vi "SetOutputVoltage.vi"(8 "error in (no error)":errorcluster, 10 "Voltage":dbl, 11 "RMXPowerSupply in":refnum<class "RMXPowerSupply.lvclass">) -> (0 "error out":errorcluster, 3 "RMXPowerSupply out":refnum<class "RMXPowerSupply.lvclass">)   [LabVIEW 2023, in "RMXPowerSupply.lvclass"]
uses:
  RMXPowerSupply.lvclass
  RMXPowerSupply.lvclass/RMXPowerSupply.ctl
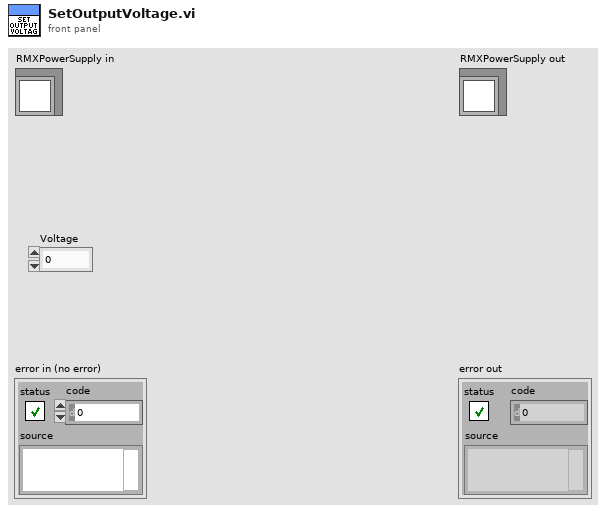
[diagram p1: front panel]
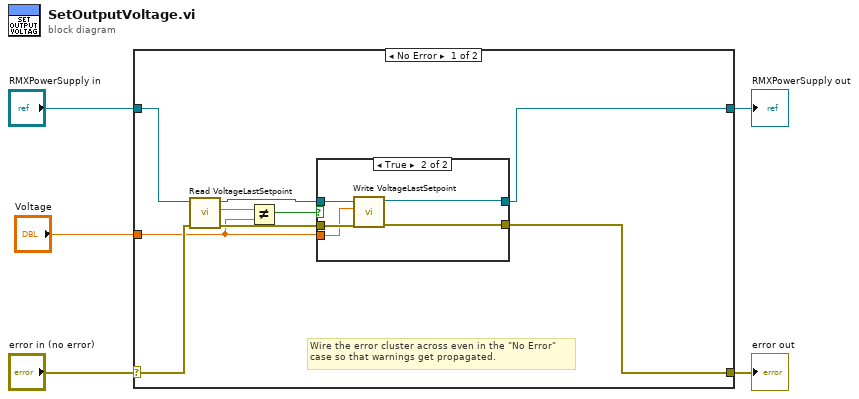
[diagram p0: block diagram]
diagram:
  n1 = case shown="No Error" "error in (no error)" {
    selector: "error in (no error)" -> [w13 w23]
    tunnel: [w7 w23] -> w4
    tunnel: [w6 w22] -> w2
    tunnel: "RMXPowerSupply in" -> [w14 w22]
    tunnel: "Voltage" -> [w8 _]
    frame No Error {
      # "Wire the error cluster across even in the \"No Error\"\ncase so that warnings get propagated."
      n2 = call-dynamic "Read VoltageLastSetpoint.vi"("error in (no error)"=w13, "RMXPowerSupply in"=w14) -> ("error out"=w10:errorcluster, "VoltageLastSetpoint"=w12:dbl, "RMXPowerSupply out"=w11:refnum<class "RMXPowerSupply.lvclass">)  [unwired: 7 in]
      n3 = Not Equal?(x=w12, y=w8) -> (x != y?=w9:bool)
      n4 = case shown="True" w9 {
        tunnel: w11 -> [w15 w21]
        tunnel: w10 -> [w16 w20]
        tunnel: w8 -> [_ w19]
        tunnel: [w16 w18] -> w7
        tunnel: [w15 w17] -> w6
        frame False {
        }
        frame True {
          n5 = call-dynamic "Write VoltageLastSetpoint.vi"("error in (no error)"=w20, "VoltageLastSetpoint"=w19, "RMXPowerSupply in"=w21) -> ("error out"=w18:errorcluster, "RMXPowerSupply out"=w17:refnum<class "RMXPowerSupply.lvclass">)  [unwired: 7 in]
        }
      }
    }
    frame Error {
    }
  }
  "error out" <- w4
  "RMXPowerSupply out" <- w2
